vi "SVT Intermodulation Distortion (1 Ch).vi"(0 "scaled signal [EU]":waveform(dbl), 3 "custom IMD signal":T10={"IMD type"=enum."CCIF/Twin-Tone", "low-frequency tone"=14000.0, "high-frequency tone"=15000.0, "amplitude ratio"=1.0, "maximum order"=5} {"amplitude ratio" format="%.1f"; "high-frequency tone" format="%.2f"; "low-frequency tone" format="%.2f"}, 5 "error in (no error)":errorcluster, 6 "desired units":T8, 8 "IMD standard":T9(ring)) -> (11 "detected low-frequency tone":cluster{"frequency [Hz]":dbl, "amplitude":dbl} {"amplitude" format="%.2f"; "frequency [Hz]" format="%.2f"}, 12 "unit labels":T7, 13 "detected high-frequency tone":cluster{"frequency [Hz]":dbl, "amplitude":dbl} {"amplitude" format="%.2f"; "frequency [Hz]" format="%.2f"}, 14 "magnitude spectrum":cluster{"f0":dbl, "df":dbl, "magnitude":dbl[]}(graph), 16 "IMD":dbl format="%.2f", 17 "intermodulation components":cluster{"frequency [Hz]":dbl, "amplitude":dbl}[](array[cluster]) {"amplitude" format="%.2f"; "frequency [Hz]" format="%.2f"}, 18 "spectrum info":T1={"channel name"="", "description"="", "x-axis units"=0, "spectral info"={"spectrum type"=enum."Power [Magnitude^2]", "linear/dB"=enum."linear", "window"=0, "window size"=0, "FFT size"=0}, "engineering units"=0, "custom label"="", "dB reference [EU]"=0.0, "peak units"=enum."rms", "weighting filter"=0, "spectral density?"=FALSE, "unit label"="", "spectrum skewed?"=FALSE, "complimentary spectrum units"=enum."none"} {"x-axis units" items=["Time (s)"=0, "Frequency-CB (Hz)"=1, "Frequency-CPB (Hz)"=1248, "Frequency-Arbitrary (Hz)"=2357, "Quefrency (s)"=2, "Revolutions (rev)"=3, "Order"=4, "Speed (RPM)"=11, "Speed (rad/s)"=21, "Index"=65535]; "weighting filter" items=["Linear", "A-weighting", "B-weighting", "C-weighting", "ITU-R 468-4", "Dolby", "CCITT", "C-message", "Wb", "Wc", "Wd", "We", "Wf", "Wh", "Wj", "Wk", "Wm", "AES17 20 kHz lowpass", "AES17 40 kHz lowpass", "AES17 20 kHz highpass", "AES17 40 kHz highpass"]; "dB reference [EU]" format="%.2f"; "engineering units" items=["custom..."=0, "V"=1, "A"=21, "C"=30, "pC"=31, "s"=32, "-"=29, "Pa"=2, "N"=20, "g"=3, "m/s^2"=4, "m/s"=5, "m"=6, "mm/s"=12, "mm"=13, "micron/s"=14, "micron"=15, "in/s^2"=7, "in/s"=8, "in"=9, "mil/s"=10, "mil"=11, "rad/s^2"=16, "rad/s"=17, "rad"=18, "deg/s^2"=26, "deg/s"=27, "deg"=28, "RPM"=22, "cycle/s^2"=23, "Hz"=24, "cycle"=25, "strain"=19]; "spectral info"."window" items=["None "=0, "Hanning"=1, "Hamming"=2, "Blackman-Harris"=3, "Exact Blackman"=4, "Blackman"=5, "Flat Top"=6, "4 Term B-Harris "=7, "7 Term B-Harris"=8, "Low Sidelobe"=9, "Force - Exponential"=10, "Gaussian"=62]}, 19 "error out":errorcluster)   [LabVIEW 2017, in "SoundVib_Distortion.lvlib"]
doc: "Computes the total intermodulation distortion and the intermodulation components based on <B>scaled signal [EU]</B> and <B>IMD standard</B>."
uses:
  <vilib>/addons/Sound and Vibration/svt_Distortion/SoundVib_Distortion.lvlib
  <vilib>/addons/_NISVFA/_Shared subVIs/Controls/svc_Spectrum Info.ctl
  <vilib>/addons/_NISVFA/_Shared subVIs/Controls/svc_X-Axis Units.ctl
  <vilib>/addons/_NISVFA/_Shared subVIs/Controls/svc_Spectrum Type.ctl
  <vilib>/addons/_NISVFA/_Shared subVIs/Controls/svc_Engineering Units Text Ring.ctl
  <vilib>/addons/_NISVFA/_Shared subVIs/Controls/svc_Weighting Filter Text Ring.ctl
  <vilib>/addons/_NISVFA/_Shared subVIs/Controls/svc_Complimentary Spectrum Units.ctl
  <vilib>/addons/_NISVFA/_Shared subVIs/Controls/svc_Window.ctl
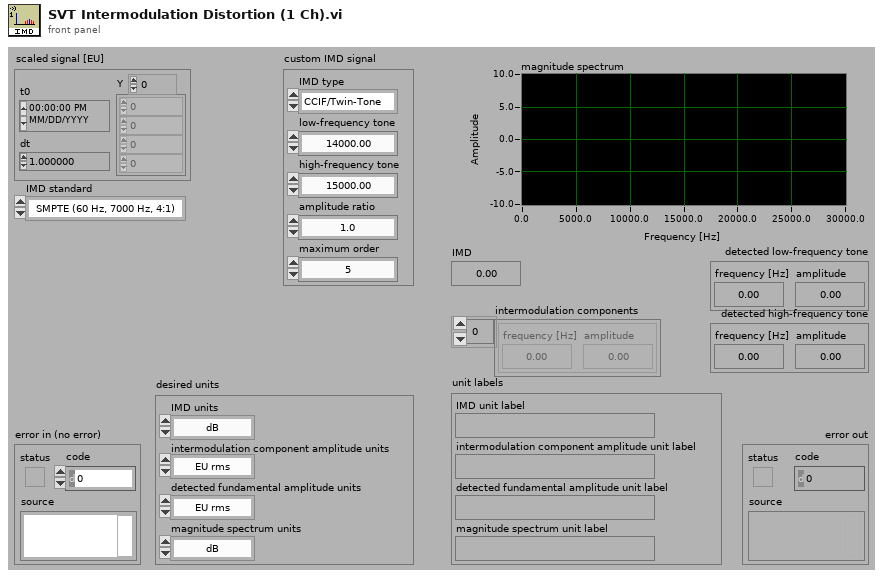
[diagram p1: front panel]
types:
  T1 = typedef "svc_Spectrum Info.ctl" = cluster{"channel name":string, "description":string, "x-axis units":T2, "spectral info":cluster{"spectrum type":T3, "linear/dB":enum16{"linear", "dB"}, "window":u16, "window size":i32, "FFT size":i32}, "engineering units":T4, "custom label":string, "dB reference [EU]":dbl, "peak units":enum16{"rms", "peak", "peak-peak"}, "weighting filter":T5, "spectral density?":bool, "unit label":string, "spectrum skewed?":bool, "complimentary spectrum units":T6}
  T2 = typedef "svc_X-Axis Units.ctl" = u16
  T3 = typedef "svc_Spectrum Type.ctl" = enum16{"FFT Spectrum [complex]", "Amplitude [Magnitude]", "Power [Magnitude^2]", "Cross Spectrum [complex]", "Frequency Response [Complex]"}
  T4 = typedef "svc_Engineering Units Text Ring.ctl" = u16
  T5 = typedef "svc_Weighting Filter Text Ring.ctl" = u16
  T6 = typedef "svc_Complimentary Spectrum Units.ctl" = enum16{"none", "radians", "degrees", "cycles", "imaginary"}
  T7 = cluster{"IMD unit label":string, "intermodulation component amplitude unit label":string, "detected fundamental amplitude unit label":string, "magnitude spectrum unit label":string}
  T8 = cluster{"IMD units":enum16{"dB", "linear ratio", "%"}, "intermodulation component amplitude units":enum16{"EU rms", "EU peak", "EU peak-peak"}, "detected fundamental amplitude units":enum16{"EU rms", "EU peak", "EU peak-peak"}, "magnitude spectrum units":enum16{"dB", "linear"}}
  T9 = enum16{"SMPTE (60 Hz, 7000 Hz, 4:1)", "DIN (250 Hz, 8000 Hz, 4:1)", "CCIF (11 kHz, 12 kHz, 1:1)", "CCIF (19 kHz, 20 kHz, 1:1)", "Custom"}
  T10 = cluster{"IMD type":enum16{"SMPTE/DIN", "CCIF/Twin-Tone"}, "low-frequency tone":dbl, "high-frequency tone":dbl, "amplitude ratio":dbl, "maximum order":i32}
  T11 = cluster{"dB On (F)":bool, "unwrap phase (F)":bool, "convert to degree (T)":bool}
  T12 = cluster{"unit label":string, "unit label":string, "unit label":string, "unit label [mag or real]":string}
  T13 = typedef "svc_Window.ctl" = u32
  T14 = enum16{"none", "input signal", "detected signal", "residual signal"}
  T15 = cluster{"complex spectrum response":cluster{"f0":dbl, "df":dbl, "complex spectrum":cdb[]}, "spectrum info":T1}
  T16 = cluster{"f0":dbl, "df":dbl, "complex spectrum":cdb[]}
  T17 = cluster{"frequency [Hz]":dbl, "converted peak amplitude":dbl}
  T18 = cluster{"detected frequency":dbl, "detected amplitude":dbl}
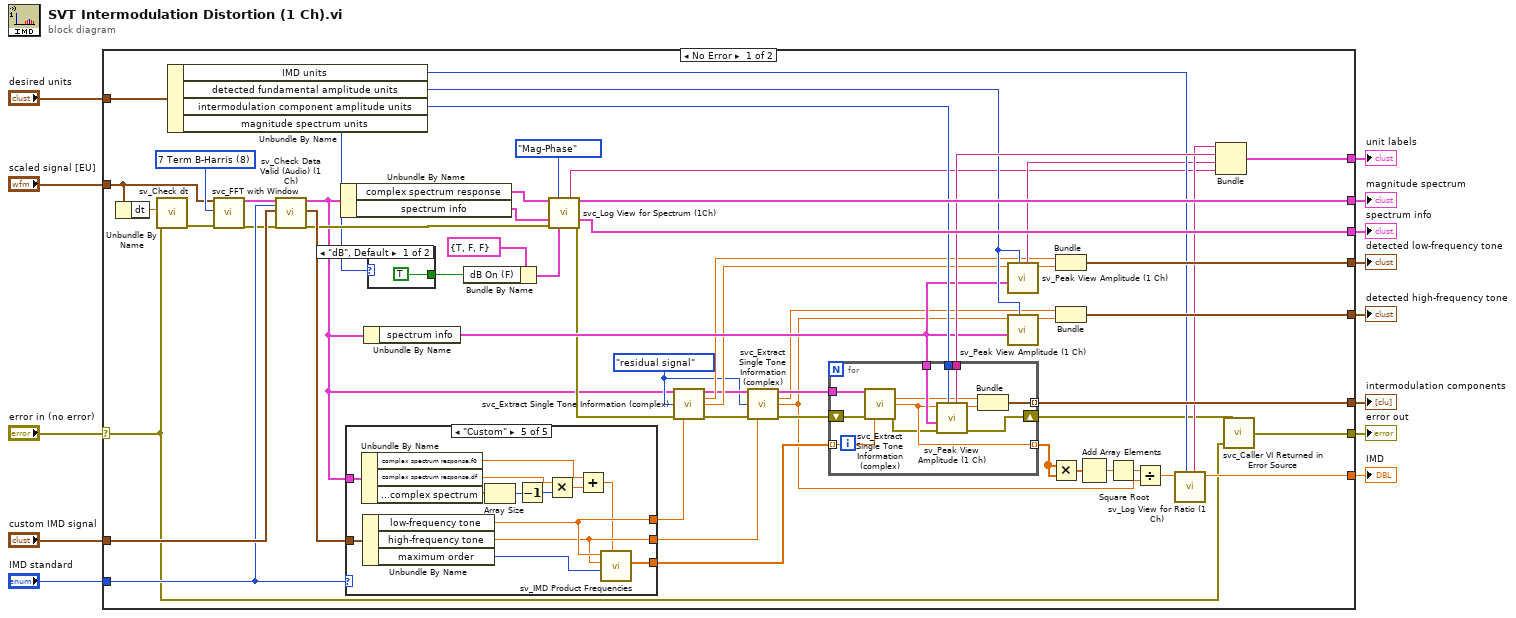
[diagram p0: block diagram]
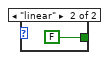
[diagram p2: hidden frame]
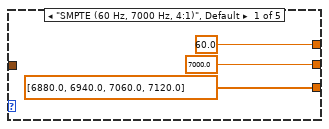
[diagram p3: hidden frame]
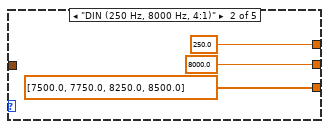
[diagram p4: hidden frame]
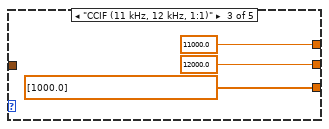
[diagram p5: hidden frame]
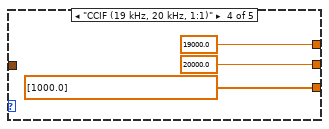
[diagram p6: hidden frame]
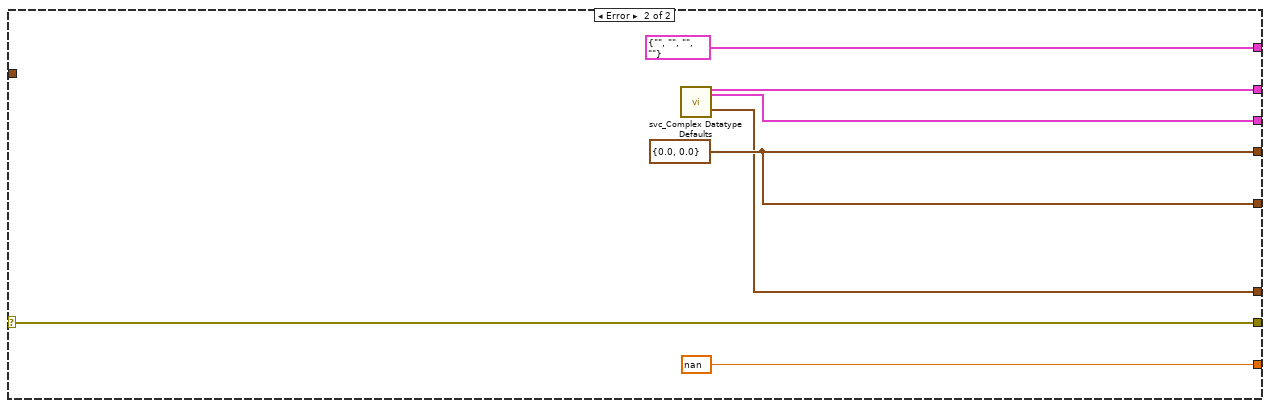
[diagram p7: hidden frame]
diagram:
  n1 = case shown="No Error" "error in (no error)" {
    selector: "error in (no error)" -> [w14 w116]
    tunnel: [w55 nan] -> w13
    tunnel: "IMD standard" -> [w46 _]
    tunnel: [w69 w114] -> w11
    tunnel: [w68 w114] -> w10
    tunnel: "scaled signal [EU]" -> [w18 _]
    tunnel: [w67 w110] -> w8
    tunnel: [w60 w112] -> w7
    tunnel: [w43 w116] -> w6
    tunnel: [w59 w111] -> w4
    tunnel: "desired units" -> [w66 _]
    tunnel: "custom IMD signal" -> [w48 _]
    tunnel: [w51 T12 {"unit label"="", "unit label"="", "unit label"="", "unit label [mag or real]"=""}] -> w1
    frame No Error {
      w36 = T13 8 items=["None ", "Hanning", "Hamming", "Blackman-Harris", "Exact Blackman", "Blackman", "Flat Top", "4 Term B-Harris ", "7 Term B-Harris", "Low Sidelobe"] ("window")
      w32 = T14."residual signal" ("export signals")
      n2 = Unbundle By Name(w18) -> ("dt"=w19:dbl)
      n3 = call <vilib>:"sv_Check dt.vi"("error in"=w14, "dt"=w19) -> ("error out"=w50:errorcluster)  [unwired: 8 in, 1 out]
      n4 = Unbundle By Name(w66) -> ("IMD units"=w52:enum16{"dB", "linear ratio", "%"}, "detected fundamental amplitude units"=w39:enum16{"EU rms", "EU peak", "EU peak-peak"}, "intermodulation component amplitude units"=w56:enum16{"EU rms", "EU peak", "EU peak-peak"}, "magnitude spectrum units"=w21:enum16{"dB", "linear"})
      n5 = call <vilib>:"svc_FFT with Window.vi"("time signal in [EU]"=w18, "window"=w36, "error in (no error)"=w50) -> ("complex spectrum"=w49:T15, "error out"=w44:errorcluster)  [unwired: 15 in]
      n6 = call <vilib>:"sv_Check Data Valid (Audio) (1 Ch).vi"("complex spectrum"=w49, "IMD standard"=w46, "custom IMD signal"=w48, "error in (no error)"=w44) -> ("complex spectrum"=w17:T15, "dup custom IMD signal"=w47:T10, "error out"=w45:errorcluster)  [unwired: 8 in, 5 out]
      n7 = Unbundle By Name(w17) -> ("complex spectrum response"=w16:T16, "spectrum info"=w15:T1)
      n8 = case shown="\"Custom\"" w46 {
        tunnel: [60.0 ("approx. fund. freq. (optional)") 250.0 ("approx. fund. freq. (optional)") 11000.0 ("approx. fund. freq. (optional)") 19000.0 ("approx. fund. freq. (optional)") w97] -> w25
        tunnel: [dbl[] [6880.0, 6940.0, 7060.0, 7120.0] ("IMD product frequencies") dbl[] [7500.0, 7750.0, 8250.0, 8500.0] ("IMD product frequencies") dbl[] [1000.0] ("IMD product frequencies") dbl[] [1000.0] ("IMD product frequencies") w96] -> w70
        tunnel: [7000.0 ("approx. fund. freq. (optional)") 8000.0 12000.0 ("approx. fund. freq. (optional)") 20000.0 ("approx. fund. freq. (optional)") w95] -> w24
        tunnel: w47 -> [_ _ _ _ w94]
        tunnel: w17 -> [_ _ _ _ w90]
        frame "SMPTE (60 Hz, 7000 Hz, 4:1)", Default {
        }
        frame "DIN (250 Hz, 8000 Hz, 4:1)" {
        }
        frame "CCIF (11 kHz, 12 kHz, 1:1)" {
        }
        frame "CCIF (19 kHz, 20 kHz, 1:1)" {
        }
        frame "Custom" {
          n9 = Unbundle By Name(w90) -> ("complex spectrum response.f0"=w88:dbl, "complex spectrum response.df"=w86:dbl, "complex spectrum response.complex spectrum"=w91:cdb[])
          n10 = Unbundle By Name(w94) -> ("low-frequency tone"=w97:dbl, "high-frequency tone"=w95:dbl, "maximum order"=w85:i32)
          n11 = Array Size(array=w91) -> (size(s)=w93:i32)
          n12 = Decrement(x=w93) -> (x-1=w87:i32)
          n13 = Multiply(x=w86, y=w87) -> (x*y=w92:dbl)
          n14 = Add(x=w88, y=w92) -> (x+y=w89:dbl)
          n15 = call <vilib>:"sv_IMD Product Frequencies.vi"("measurement bandwidth"=w89, "override order"=w85, "f2"=w95, "f1"=w97) -> ("IMD product frequencies"=w96:dbl[])  [unwired: 5 in, 2 out]
        }
      }
      n16 = Unbundle By Name(w17) -> ("spectrum info"=w38:T1)
      n17 = case shown="\"dB\", Default" w21 {
        tunnel: [TRUE ("dB On (F)") FALSE ("dB On (F)")] -> w65
        frame "dB", Default {
        }
        frame "linear" {
        }
      }
      n18 = Bundle By Name(cluster=T11 {"dB On (F)"=TRUE, "unwrap phase (F)"=FALSE, "convert to degree (T)"=FALSE} ("view"), "dB On (F)"=w65) -> (w23:T11)
      n19 = call <vilib>:"svc_Log View for Spectrum (1Ch).vi"("complex spectrum"=w16, "View"=enum16{"Mag-Phase", "Real-Imaginary"}."Mag-Phase" ("output spectrum type"), "spectrum info in"=w15, "error in (no error)"=w45, "view"=w23) -> ("unit label [mag or real]"=w22:string, "magnitude or real"=w59:cluster{"f0":dbl, "df":dbl, dbl[]}, "spectrum info out"=w60:T1, "error out"=w30:errorcluster)  [unwired: 5 in, 2 out]
      n20 = call <vilib>:"svc_Extract Single Tone Information (complex).vi"("complex spectrum"=w17, "export signals"=w32, "error in"=w30, "approximate frequency [Hz]"=w25) -> ("complex spectrum"=w33:T15, "frequency [Hz]"=w35:dbl, "amplitude [EU pk]"=w34:dbl, "error out"=w31:errorcluster)  [unwired: 6 in, 2 out]
      n21 = call <vilib>:"svc_Extract Single Tone Information (complex).vi"("complex spectrum"=w33, "export signals"=w32, "error in"=w31, "approximate frequency [Hz]"=w24) -> ("complex spectrum"=w28:T15, "frequency [Hz]"=w27:dbl, "amplitude [EU pk]"=w26:dbl, "error out"=w29:errorcluster)  [unwired: 6 in, 2 out]
      n22 = for {
        shift-right: [w104] -> w37
        shift-left: w29 -> [w100]
        tunnel: w70 -> [w98] mode=indexing
        tunnel: [w101] -> w62 mode=indexing
        tunnel: [w109] -> w67 mode=indexing
        tunnel: w56 -> [w107]
        tunnel: [w108] -> w54
        tunnel: w38 -> [w105]
        tunnel: w28 -> [w103]
        n23 = call <vilib>:"svc_Extract Single Tone Information (complex).vi"("complex spectrum"=w103, "error in"=w100, "approximate frequency [Hz]"=w98) -> ("frequency [Hz]"=w102:dbl, "amplitude [EU pk]"=w101:dbl, "error out"=w99:errorcluster)  [unwired: 7 in, 3 out]
        n24 = call <vilib>:"sv_Peak View Amplitude (1 Ch).vi"("peak units"=w107, "error in (no error)"=w99, "spectrum info"=w105, "peak amplitude [EU pk]"=w101) -> ("error out"=w104:errorcluster, "converted peak amplitude"=w106:dbl, "unit label"=w108:string)  [unwired: 5 in]
        n25 = Bundle("frequency [Hz]"=w102, "converted peak amplitude"=w106) -> (w109:T17)  [unwired: 1 in]
      }
      n26 = call <vilib>:"sv_Peak View Amplitude (1 Ch).vi"("peak units"=w39, "spectrum info"=w38, "peak amplitude [EU pk]"=w34) -> ("converted peak amplitude"=w57:dbl, "unit label"=w40:string)  [unwired: 6 in, 1 out]
      n27 = call <vilib>:"sv_Peak View Amplitude (1 Ch).vi"("peak units"=w39, "spectrum info"=w38, "peak amplitude [EU pk]"=w26) -> ("converted peak amplitude"=w58:dbl)  [unwired: 6 in, 2 out]
      n28 = Multiply(x=w62, y=w62) -> (x*y=w64:dbl[])
      n29 = Bundle("frequency [Hz]"=w35, "converted peak amplitude"=w57) -> (w68:T17)  [unwired: 1 in]
      n30 = Bundle("frequency [Hz]"=w27, "converted peak amplitude"=w58) -> (w69:T17)  [unwired: 1 in]
      n31 = Add Array Elements(numeric array=w64) -> (sum=w63:dbl)
      n32 = Square Root(x=w63) -> (sqrt(x)=w42:dbl)
      n33 = Divide(x=w42, y=w26) -> (x/y=w41:dbl)
      n34 = call <vilib>:"sv_Log View for Ratio (1 Ch).vi"("ratio units"=w52, "linear ratio"=w41) -> ("converted ratio"=w55:dbl, "unit label"=w53:string)  [unwired: 7 in, 1 out]
      n35 = Bundle("unit label"=w53, "unit label"=w54, "unit label"=w40, "unit label [mag or real]"=w22) -> (w51:T12)  [unwired: 1 in]
      n36 = call <vilib>:"svc_Caller VI Returned in Error Source.vi"("warning input to caller"=w14, "error in (no error)"=w37) -> ("error out"=w43:errorcluster)  [unwired: 3 in]
    }
    frame Error {
      w114 = T18 {"detected frequency"=0.0, "detected amplitude"=0.0}
      n37 = call <vilib>:"svc_Complex Datatype Defaults.vi"() -> ("empty spectrum"=w111:cluster{"f0":dbl, "df":dbl, "magnitude":dbl[]}, "dead spectrum info"=w112:T1, "empty array of peaks"=w110:cluster{"frequency":dbl, "value":dbl}[])  [unwired: 11 in, 6 out]
    }
  }
  "error out" <- w6
  "IMD" <- w13
  "intermodulation components" <- w8
  "unit labels" <- w1
  "spectrum info" <- w7
  "detected low-frequency tone" <- w10
  "detected high-frequency tone" <- w11
  "magnitude spectrum" <- w4
